vi "Valid.vi"(8 "error in (no error)":errorcluster, 11 "BetterHandle In":refnum<class "BetterHandle.lvclass">) -> (0 "error out":errorcluster, 2 "Valid handle?":bool, 3 "BetterHandle Out":refnum<class "BetterHandle.lvclass">)   [LabVIEW 2020, in "BetterDragAndDrop.lvlib" / "BetterHandle.lvclass"]
uses:
  BetterHandle.lvclass
  BetterHandle.lvclass/BetterHandle.ctl
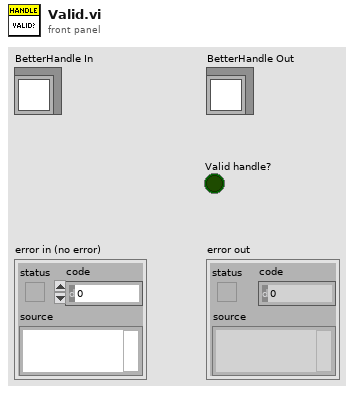
[diagram p1: front panel]
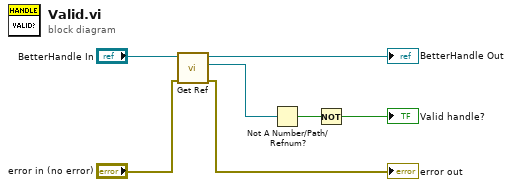
[diagram p0: block diagram]
diagram:
  n1 = call-dynamic "Get Ref.vi"("error in (no error)"="error in (no error)", "BetterHandle in"="BetterHandle In") -> ("error out"=→"error out":errorcluster, "Tree/LB/MCL ref"=w5:refnum<vi>, "BetterHandle out"=→"BetterHandle Out":refnum<class "BetterHandle.lvclass">)  [unwired: 7 in]
  n2 = Not A Number/Path/Refnum?(number/path/refnum=w5) -> (NaN/Path/Refnum?=w4:bool)
  n3 = Not(x=w4) -> (.not. x?=→"Valid handle?":bool)
